vi "Extras_1SDI.vi"(8 "Scope+Safety":T3={"Safety First"={"lim reset"=FALSE, "no limit"=FALSE, "pos slew rate * dt"=100, "neg slew rate * dt"=-100, "Count(Ticks)"=0}, "Scope IPs"={"Trigger Direction"=enum."minus-plus", "Trigger Delay (ms)"=0.0, "Aquisition Rate (kHz)"=4000.0, "Trigger Offset (V)"=0.0, "Scale Offset"={"Scaling"={"Error signal"=1, "Output"=1, "DC Monitor"=1, "Threshold"=1}, "Offset"={"Error Signal"=0, "Output"=0, "DC Monitor"=0, "Threshold"=0}}}}, 11 "Extras 1SDI":T4={"Error Bit Shift "={"EPR BS"=0, "HD A x"=0, "HD A p"=0, "HD B x"=0, "HD B p"=0}, "I Max value"=20000, "Scan Offset"={"EPR BS"=0.0, "HD A"=0.0, "HD B"=0.0}, "Scan Ampl."={"EPR BS"=0.0, "HD A"=0.0, "HD B"=0.0}, "Scan-PII thresh"={"EPR BS"=0, "Homodyne A"=0, "Homodyne B"=0}, "Re-Scan thresh"={"EPR BS"=1000, "Homodyne A"=1000, "Homodyne B"=1000}, "Post-Offset"={"HD A x"=0.0, "HD A p"=0.0, "HD B x"=0.0, "HD B p"=0.0}}) -> (0 "Extras Homodyne B":T1, 1 "Extras Homodyne A":T1, 3 "Extras EPR BS":T2)   [LabVIEW 2011]
uses:
  Strict Type Defs/Extras 1SDI.ctl
  Strict Type Defs/Double ISDI control.ctl
  Strict Type Defs/I16 1SDI Control.ctl
  Strict Type Defs/Scope and Safety.ctl
  Strict Type Defs/Extras PII 1SDI.ctl
  Strict Type Defs/Extras PII 1SDI HD.ctl
panel:
  in  "Extras HD_1SDI":T1
  in  "Extras HD 1SDI":T1
  in  "Extras PII 1SDI":T2
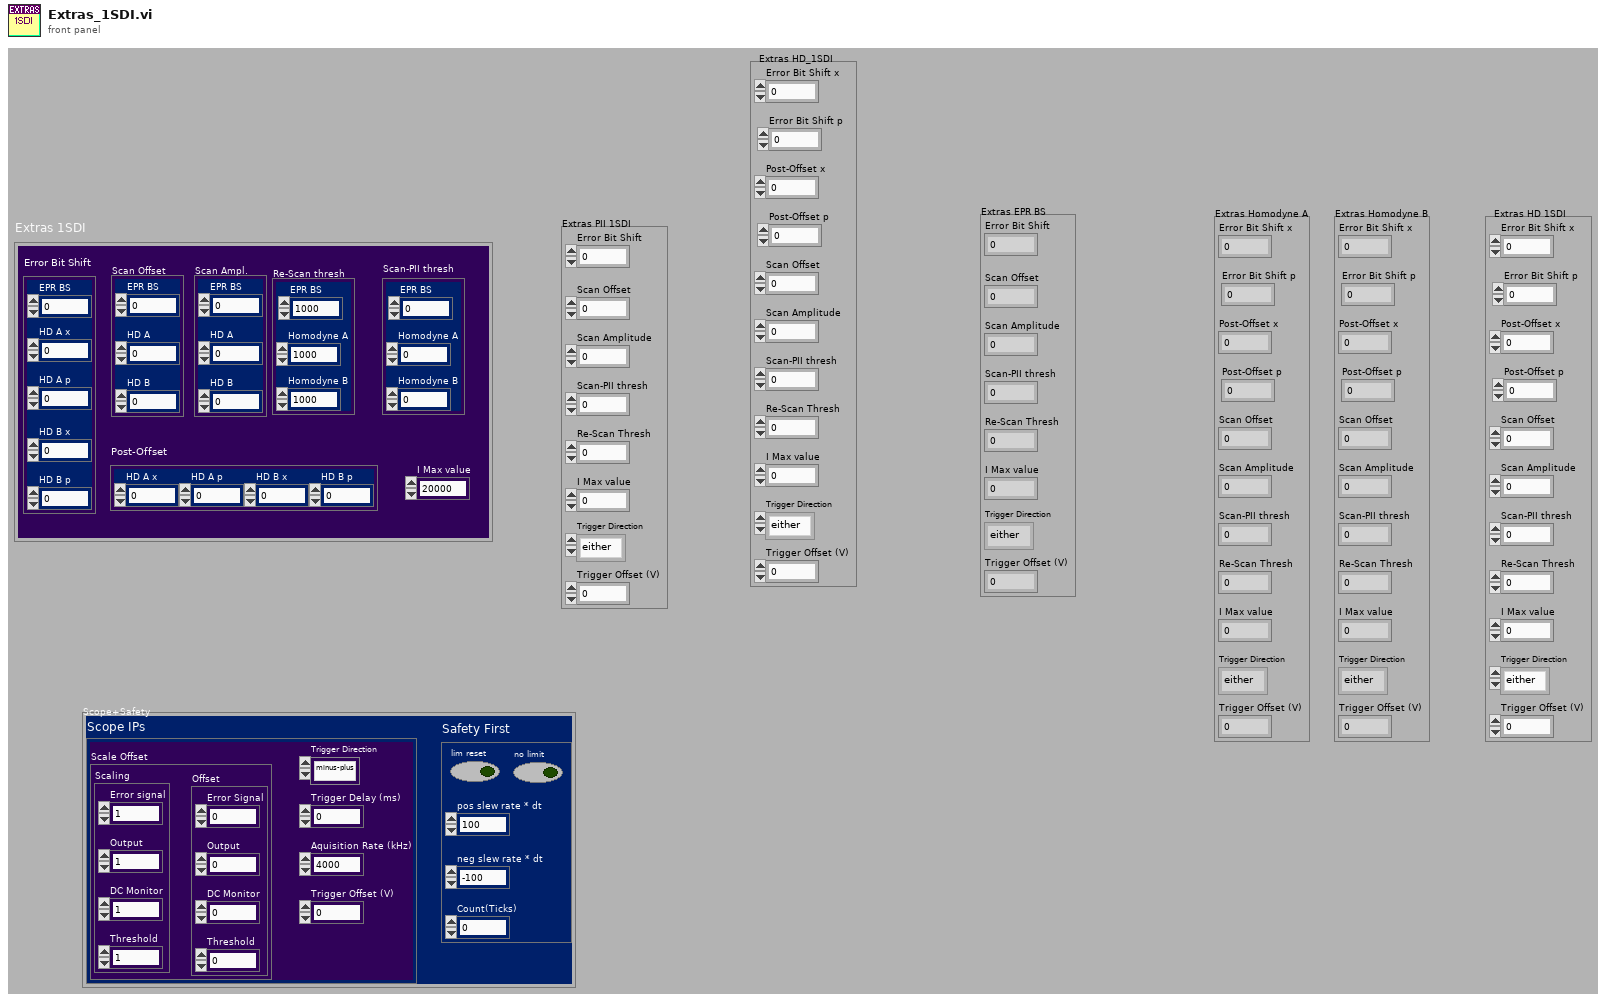
[diagram p1: front panel]
types:
  T1 = typedef "Extras PII 1SDI HD.ctl" = cluster{"Error Bit Shift p":i16, "Scan Offset":dbl, "Scan Amplitude":dbl, "Scan-PII thresh":i16, "Re-Scan Thresh":i16, "I Max value":i32, "Trigger Direction":enum8{"either", "minus-plus", "plus-minus"}, "Trigger Offset (V)":dbl, "Error Bit Shift x":i16, "Post-Offset p":dbl, "Post-Offset x":dbl}
  T2 = typedef "Extras PII 1SDI.ctl" = cluster{"Error Bit Shift":i16, "Scan Offset":dbl, "Scan Amplitude":dbl, "Scan-PII thresh":i16, "Re-Scan Thresh":i16, "I Max value":i32, "Trigger Direction":enum8{"either", "minus-plus", "plus-minus"}, "Trigger Offset (V)":dbl}
  T3 = typedef "Scope and Safety.ctl" = cluster{"Safety First":cluster{"lim reset":bool, "no limit":bool, "pos slew rate * dt":i16, "neg slew rate * dt":i16, "Count(Ticks)":u32}, "Scope IPs":cluster{"Trigger Direction":enum8{"either", "minus-plus", "plus-minus"}, "Trigger Delay (ms)":dbl, "Aquisition Rate (kHz)":dbl, "Trigger Offset (V)":dbl, "Scale Offset":cluster{"Scaling":cluster{"Error signal":i16, "Output":i16, "DC Monitor":i16, "Threshold":i16}, "Offset":cluster{"Error Signal":i16, "Output":i16, "DC Monitor":i16, "Threshold":i16}}}}
  T4 = typedef "Extras 1SDI.ctl" = cluster{"Error Bit Shift ":cluster{"EPR BS":i16, "HD A x":i16, "HD A p":i16, "HD B x":i16, "HD B p":i16}, "I Max value":i32, "Scan Offset":T5, "Scan Ampl.":T5, "Scan-PII thresh":T6, "Re-Scan thresh":T6, "Post-Offset":cluster{"HD A x":dbl, "HD A p":dbl, "HD B x":dbl, "HD B p":dbl}}
  T5 = typedef "Double ISDI control.ctl" = cluster{"EPR BS":dbl, "HD A":dbl, "HD B":dbl}
  T6 = typedef "I16 1SDI Control.ctl" = cluster{"EPR BS":i16, "Homodyne A":i16, "Homodyne B":i16}
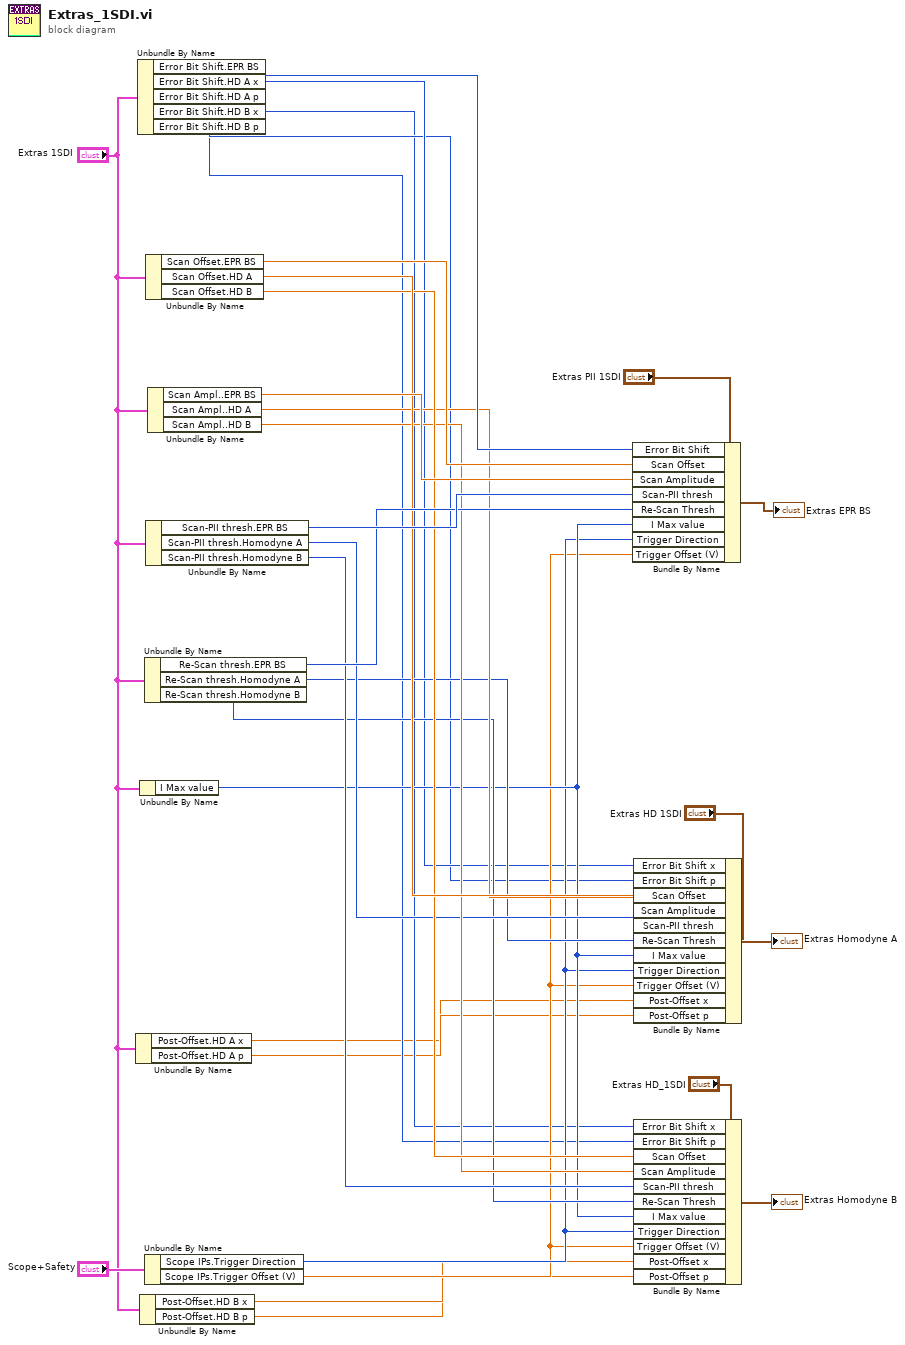
[diagram p0: block diagram]
diagram:
  n1 = Unbundle By Name("Extras 1SDI") -> ("Post-Offset.HD A x"=w6:dbl, "Post-Offset.HD A p"=w7:dbl)
  n2 = Unbundle By Name("Extras 1SDI") -> ("Error Bit Shift.EPR BS"=w30:i16, "Error Bit Shift.HD A x"=w11:i16, "Error Bit Shift.HD A p"=w10:i16, "Error Bit Shift.HD B x"=w9:i16, "Error Bit Shift.HD B p"=w8:i16)
  n3 = Unbundle By Name("Extras 1SDI") -> ("I Max value"=w15:i32)
  n4 = Unbundle By Name("Extras 1SDI") -> ("Post-Offset.HD B x"=w4:dbl, "Post-Offset.HD B p"=w3:dbl)
  n5 = Unbundle By Name("Extras 1SDI") -> ("Re-Scan thresh.EPR BS"=w26:i16, "Re-Scan thresh.Homodyne A"=w17:i16, "Re-Scan thresh.Homodyne B"=w16:i16)
  n6 = Unbundle By Name("Scope+Safety") -> ("Scope IPs.Trigger Direction"=w14:enum8{"either", "minus-plus", "plus-minus"}, "Scope IPs.Trigger Offset (V)"=w13:dbl)
  n7 = Unbundle By Name("Extras 1SDI") -> ("Scan Offset.EPR BS"=w29:dbl, "Scan Offset.HD A"=w23:dbl, "Scan Offset.HD B"=w22:dbl)
  n8 = Unbundle By Name("Extras 1SDI") -> ("Scan-PII thresh.EPR BS"=w27:i16, "Scan-PII thresh.Homodyne A"=w19:i16, "Scan-PII thresh.Homodyne B"=w18:i16)
  n9 = Unbundle By Name("Extras 1SDI") -> ("Scan Ampl..EPR BS"=w28:dbl, "Scan Ampl..HD A"=w21:dbl, "Scan Ampl..HD B"=w20:dbl)
  n10 = Bundle By Name(cluster="Extras PII 1SDI", "Error Bit Shift"=w30, "Scan Offset"=w29, "Scan Amplitude"=w28, "Scan-PII thresh"=w27, "Re-Scan Thresh"=w26, "I Max value"=w15, "Trigger Direction"=w14, "Trigger Offset (V)"=w13) -> (→"Extras EPR BS":T2)
  n11 = Bundle By Name(cluster="Extras HD 1SDI", "Error Bit Shift x"=w11, "Error Bit Shift p"=w10, "Scan Offset"=w23, "Scan Amplitude"=w21, "Scan-PII thresh"=w19, "Re-Scan Thresh"=w17, "I Max value"=w15, "Trigger Direction"=w14, "Trigger Offset (V)"=w13, "Post-Offset x"=w6, "Post-Offset p"=w7) -> (→"Extras Homodyne A":T1)
  n12 = Bundle By Name(cluster="Extras HD_1SDI", "Error Bit Shift x"=w9, "Error Bit Shift p"=w8, "Scan Offset"=w22, "Scan Amplitude"=w20, "Scan-PII thresh"=w18, "Re-Scan Thresh"=w16, "I Max value"=w15, "Trigger Direction"=w14, "Trigger Offset (V)"=w13, "Post-Offset x"=w4, "Post-Offset p"=w3) -> (→"Extras Homodyne B":T1)
